vi "execute_clamp_protocol_v02.vi"(4 "number of samples per channel":i32=-1, 6 "command data in":dbl[](array[numeric]) format="%0.2f", 7 "which clamp":enum16{"VClamp", "IClamp"}(ring), 8 "error in":errorcluster, 9 "AO in":refnum<k21>, 11 "AI in":refnum<k21>) -> (0 "error out":errorcluster, 1 "AO out":refnum<k21>, 2 "output Graph":waveform(dbl)(graph), 3 "AI out":refnum<k21>)   [LabVIEW 2015]
uses:
  <vilib>/DAQmx/read.llb/DAQmx Read (Analog Wfm 1Chan NSamp).vi
  <vilib>/DAQmx/write.llb/DAQmx Write (Analog 1D DBL 1Chan NSamp).vi
panel:
  out "number of samples written per channel":u32
  # "EXECUTE CLAMP PROTOCOL"
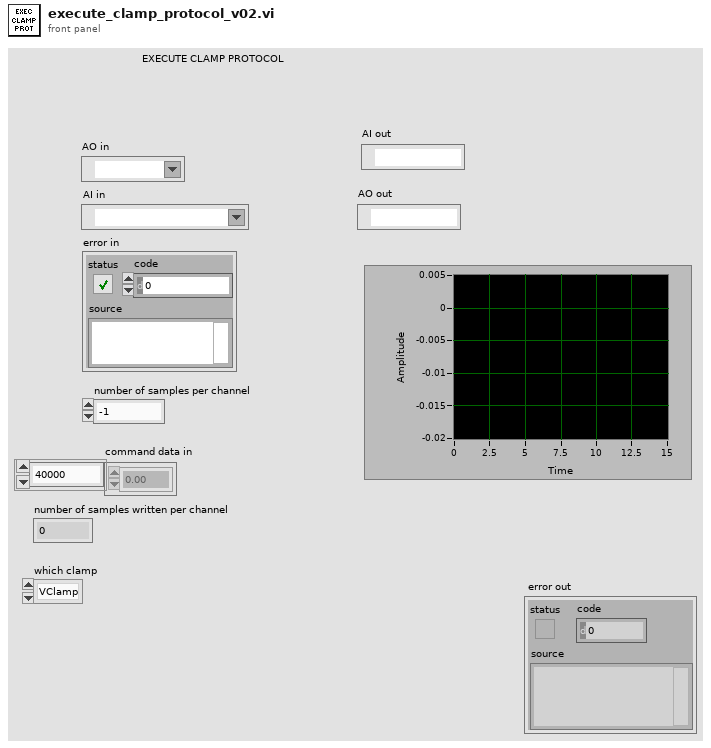
[diagram p1: front panel]
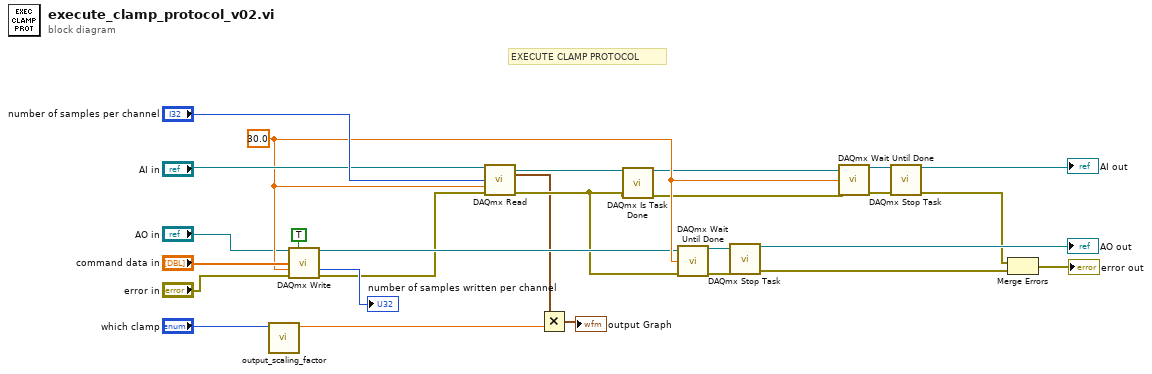
[diagram p0: block diagram]
diagram:
  w13 = 30.0 ("timeout (sec)")
  # "EXECUTE CLAMP PROTOCOL"
  n1 = call "output_scaling_factor.vi"("which clamp"="which clamp") -> ("output scaling factor"=w1:dbl)  [unwired: 10 in]
  n2 = call-poly <vilib>:"DAQmx Write.vi"("task/channels in"="AO in", "auto start"=TRUE, "data"="command data in", "timeout"=w13, "error in"="error in") -> ("task out"=w8:refnum<k21>, "number of samples written per channel"=→"number of samples written per channel":u32, "error out"=w6:errorcluster)  [unwired: 8 in]
  n3 = call-poly <vilib>:"DAQmx Read.vi"("task/channels in"="AI in", "number of samples per channel"="number of samples per channel", "timeout"=w13, "error in"=w6) -> ("task out"=w11:refnum<k21>, "data"=w3:waveform(dbl), "error out"=w7:errorcluster)  [unwired: 9 in]
  n4 = Multiply(x=w3, y=w1) -> (x*y=→"output Graph":waveform(dbl))
  n5 = call <vilib>:"DAQmx Is Task Done.vi"("task/channels in"=w11, "error in"=w7) -> ("task out"=w9:refnum<k21>, "error out"=w10:errorcluster)  [unwired: 11 in, 1 out]
  n6 = call <vilib>:"DAQmx Wait Until Done.vi"("task/channels in"=w8, "timeout (sec)"=w13, "error in"=w7) -> ("task out"=w24:refnum<k21>, "error out"=w23:errorcluster)  [unwired: 11 in]
  n7 = call <vilib>:"DAQmx Stop Task.vi"("task/channels in"=w24, "error in"=w23) -> ("task out"=→"AO out":refnum<k21>, "error out"=w15:errorcluster)  [unwired: 12 in]
  n8 = call <vilib>:"DAQmx Wait Until Done.vi"("task/channels in"=w9, "timeout (sec)"=w13, "error in"=w10) -> ("task out"=w22:refnum<k21>, "error out"=w17:errorcluster)  [unwired: 11 in]
  n9 = call <vilib>:"DAQmx Stop Task.vi"("task/channels in"=w22, "error in"=w17) -> ("task out"=→"AI out":refnum<k21>, "error out"=w16:errorcluster)  [unwired: 12 in]
  n10 = Merge Errors(w16, w15) -> (→"error out":errorcluster)
